vi "Manual Catapult Mode.vi"() -> (0 "Claw?":bool, 1 "Pin Shooter?":bool, 2 "Low Power Solenoid":bool, 3 "High Power Solenoid":bool)   [LabVIEW 2015]
uses:
  Robot Global Data.vi
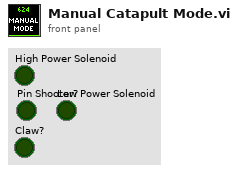
[diagram p1: front panel]
types:
  T1 = typedef "Manual Catapult Cluster.ctl" = cluster{"High Power Shot?":bool, "Shoot?":bool, "Secure Ball?":bool}
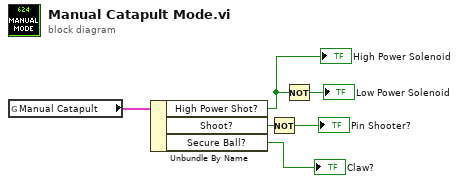
[diagram p0: block diagram]
diagram:
  n1 = global read "Robot Global Data.vi" "Manual Catapult"() -> (w6:T1)
  n2 = Unbundle By Name(w6) -> ("High Power Shot?"=w4:bool, "Shoot?"=w5:bool, "Secure Ball?"=→"Claw?":bool)
  "High Power Solenoid" <- w4
  n3 = Not(x=w5) -> (.not. x?=→"Pin Shooter?":bool)
  n4 = Not(x=w4) -> (.not. x?=→"Low Power Solenoid":bool)
